vi "Calculate Gyro Turn Setpoint.vi"(9 "End Angle":dbl) -> (1 "Turn Setpoint":dbl)   [LabVIEW 2018]
uses:
  Framework/Robot Global Data.vi
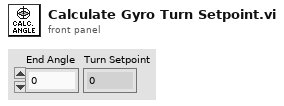
[diagram p1: front panel]
types:
  T1 = cluster{"X Angle":dbl, "Y Angle":dbl, "Z Angle":dbl}
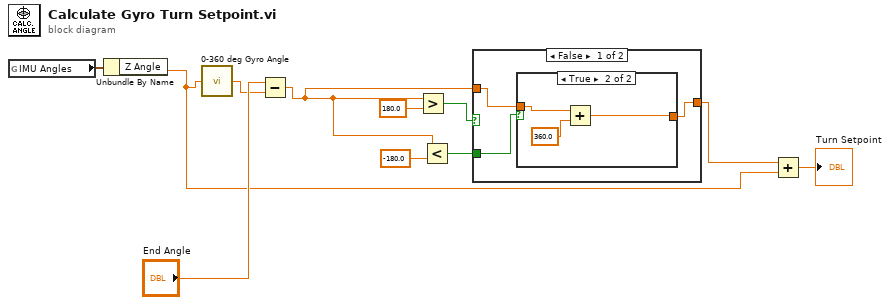
[diagram p0: block diagram]
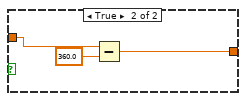
[diagram p3: hidden frame]
diagram:
  n1 = global read "Robot Global Data.vi" "IMU Angles"() -> (w10:T1)
  n2 = Unbundle By Name(w10) -> ("Z Angle"=w1:dbl)
  n3 = call "0-360 deg Gyro Angle.vi"("Raw Angle"=w1) -> ("0-360 deg Angle"=w2:dbl)
  n4 = Subtract(x="End Angle", y=w2) -> (x-y=w6:dbl)
  n5 = Greater?(x=w6, y=180.0) -> (0:w7:bool)
  n6 = Less?(x=w6, y=-180.0) -> (x < y?=w5:bool)
  n7 = case shown="False" w7 {
    tunnel: w6 -> [w13 w21]
    tunnel: [w12 w19] -> w4
    tunnel: w5 -> [w14 _]
    frame False {
      n8 = case shown="True" w14 {
        tunnel: w13 -> [w15 w18]
        tunnel: [w15 w16] -> w12
        frame False {
        }
        frame True {
          n9 = Add(x=w18, y=360.0) -> (x+y=w16:dbl)
        }
      }
    }
    frame True {
      n10 = Subtract(x=w21, y=360.0) -> (x-y=w19:dbl)
    }
  }
  n11 = Add(x=w4, y=w1) -> (x+y=→"Turn Setpoint":dbl)
